vi "Launcher.vi"() -> ()   [LabVIEW 2018, in "MonSys_Server_Actor.lvlib" / "MonSys_Server_Actor.lvclass"]
doc: "This VI is just an example and could be replaced with your application"
uses:
  MonSys_Server_Actor.lvclass
  _MonSys_LIB/OnlineData.ctl
  _MonSys_LIB/OnlineData_State.ctl
  C:/Program Files (x86)/National Instruments/LabVIEW 2018/vi.lib/ActorFramework/Actor/Actor.lvclass
  MonSys_Server_Actor Messages/Set_OnlineData Msg/Set_OnlineData Msg.lvclass/Set_OnlineData Msg.ctl
  <vilib>/ActorFramework/Message Enqueuer/Message Enqueuer.lvclass/Message Enqueuer.ctl
  MonSys_Server_Actor Messages/FrontPanel_Control Msg/FrontPanel_Control Msg.lvclass/FrontPanel_Control Msg.ctl
  <vilib>/ActorFramework/Message Enqueuer/Enqueue.vi
  MonSys_Server_Actor Messages/Set_OnlineData Msg/Set_OnlineData Msg.lvclass
  C:/Program Files (x86)/National Instruments/LabVIEW 2018/vi.lib/ActorFramework/Message/Message.lvclass
  MonSys_Server_Actor Messages/FrontPanel_Control Msg/FrontPanel_Control Msg.lvclass
  <vilib>/ActorFramework/Stop Msg/Stop Msg.lvclass
  <vilib>/ActorFramework/Message Priority Queue/Priority Enqueue.vi
  <vilib>/ActorFramework/Actor/Actor.lvclass
  _MonSys_LIB/_MonSys_LIB.lvlib
panel:
  in  "Actor_FP_control":bool
  in  "Stop":bool
  in  "Data_IN":T1={"Online"=TRUE, "Info"="", "OnlineData_State"=0} {"OnlineData_State" items=["Idle", "Manually", "Automatic"]}
  # "System: 1"
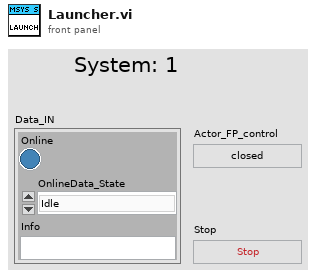
[diagram p1: front panel]
types:
  T1 = typedef "_MonSys_LIB.lvlib/OnlineData.ctl" = cluster{"Online":bool, "Info":string, "OnlineData_State":T2}
  T2 = typedef "_MonSys_LIB.lvlib/OnlineData_State.ctl" = u16
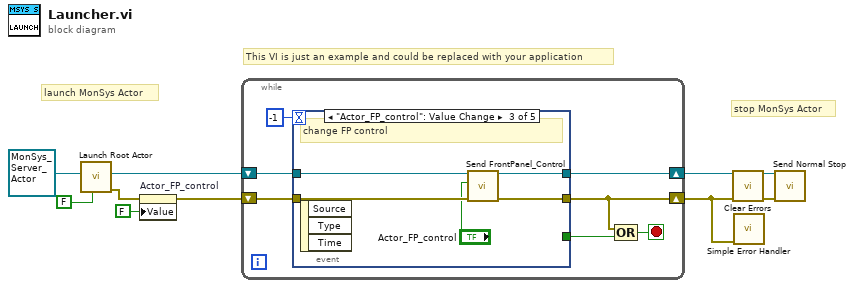
[diagram p0: block diagram]
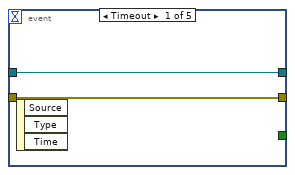
[diagram p2: hidden frame]
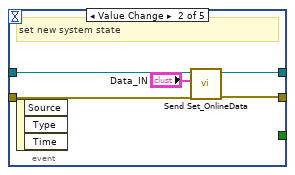
[diagram p3: hidden frame]
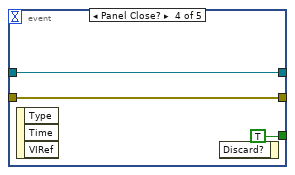
[diagram p4: hidden frame]
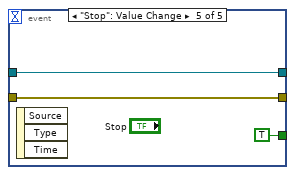
[diagram p5: hidden frame]
diagram:
  # "stop MonSys Actor"
  # "launch MonSys Actor"
  # "This VI is just an example and could be replaced with your application"
  n1 = call <vilib>:"Launch Root Actor.vi"("Open Actor Core front panel? (F)"=FALSE, "Actor"=refnum<class "MonSys_Server_Actor.lvclass"> refnum ("WebServer.lvlib:WebServer.lvclass")) -> ("error out"=w2:errorcluster, "Actor's Enqueuer"=w7:refnum<class "Message Enqueuer.lvclass">)  [unwired: 8 in]
  n2 = property on="Actor_FP_control" class="Bool (strict)"(error in=w2, "Value"=FALSE ("FP_control")) -> (error out=w1:errorcluster)  [unwired: 1 in, 1 out]
  n3 = while {
    shift-right: [w14] -> w6
    shift-left: w7 -> [w16]
    shift-right: [w10] -> w5
    shift-left: w1 -> [w12]
    stop <- w11 stop-if-true
    n4 = event shown="[2] \"Actor_FP_control\": Value Change" {
      selector: _ -> [_ _ _ _ _]
      dyn-events: _ -> [_ _ _ _ _]
      timeout: -1 -> [_ _ _ _ _]
      tunnel: w16 -> [w18 w22 w28 w30 w34]
      tunnel: [_ _ _ TRUE TRUE] -> w15
      tunnel: [w18 w21 w26 w30 w34] -> w14
      tunnel: [w17 w20 w25 w29 w33] -> w10
      tunnel: w12 -> [w17 w19 w27 w29 w33]
      event Timeout {
        n5 = event-data() -> ()  [unwired: 1 in, 3 out]
      }
      event Value Change {
        # "set new system state"
        n6 = event-data() -> ()  [unwired: 1 in, 3 out]
        n7 = call "Send Set_OnlineData.vi"("error in (no error)"=w19, "Data_IN"="Data_IN", "Message Enqueuer"=w22) -> ("error out"=w20:errorcluster, "Message Enqueuer out"=w21:refnum<class "Message Enqueuer.lvclass">)  [unwired: 7 in]
      }
      event "Actor_FP_control": Value Change {
        # "change FP control"
        n8 = event-data() -> ()  [unwired: 1 in, 3 out]
        n9 = call "Send FrontPanel_Control.vi"("error in (no error)"=w27, "FP_open?"="Actor_FP_control", "Message Enqueuer"=w28) -> ("error out"=w25:errorcluster, "Message Enqueuer out"=w26:refnum<class "Message Enqueuer.lvclass">)  [unwired: 7 in]
      }
      event Panel Close? {
        n10 = event-data() -> ()  [unwired: 1 in, 3 out]
        n11 = event-data() -> ()  [unwired: 2 in, 1 out]
      }
      event "Stop": Value Change {
        n12 = event-data() -> ()  [unwired: 1 in, 3 out]
      }
    }
    n13 = Compound Arithmetic op=OR(w10, w15) -> (w11:bool)
  }
  n14 = call <vilib>:"Clear Errors.vi"("error in (no error)"=w5) -> ("error out"=w4:errorcluster)  [unwired: 5 in, 1 out]
  n15 = call <vilib>:"Simple Error Handler.vi"("error in (no error)"=w5) -> ()  [unwired: 4 in, 5 out]
  n16 = call <vilib>:"Send Normal Stop.vi"("error in (no error)"=w4, "Message Enqueuer"=w6) -> ()  [unwired: 9 in, 1 out]
